vi "find center.vi"(3 "error in":errorcluster, 4 "Split point":dbl, 5 "Image":dbl[][](array[numeric])) -> (0 "error out":errorcluster, 1 "Y - centroid":dbl[](array[numeric]), 2 "X - centroid":dbl[](array[numeric]))   [LabVIEW 2014]
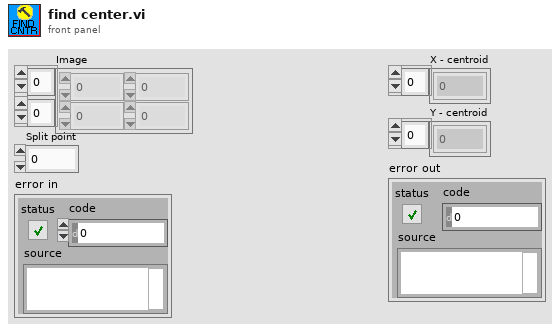
[diagram p1: front panel]
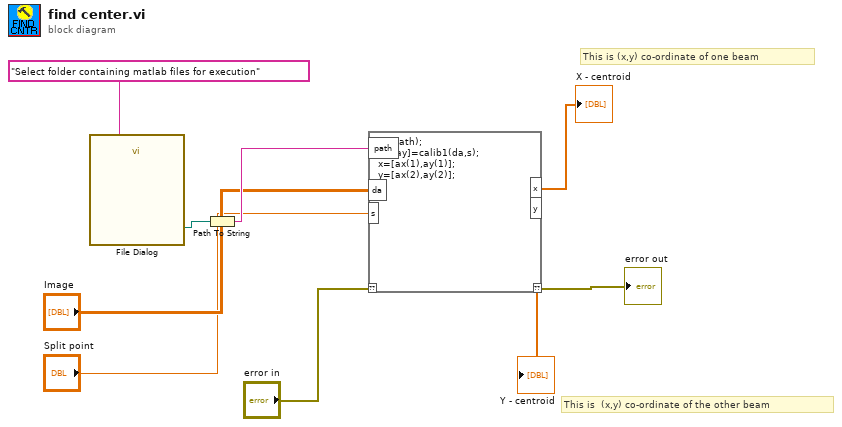
[diagram p0: block diagram]
diagram:
  # "This is  (x,y) co-ordinate of the other beam"
  # "This is (x,y) co-ordinate of one beam"
  n1 = call "File Dialog"("prompt"="Select folder containing matlab files for execution") -> ("selected path"=w9:path)  [unwired: 11 in, 3 out]
  n2 = Path To String(path=w9) -> (string=w8:string)
  n3 = script code="cd(path);\n[ax,ay]=calib1(da,s);\nx=[ax(1),ay(1)];\ny=[ax(2),ay(2)];"("??"="error in", "path"=w8, "da"="Image", "s"="Split point") -> ("??"=→"error out":errorcluster, "x"=→"X - centroid":dbl[], "y"=→"Y - centroid":dbl[])
